vi "Config Core.vi"(8 "Error In":errorcluster, 10 "IConfigIn":refnum<class "IConfig.lvclass">, 11 "HardwareIn":refnum<class "IReference.lvclass">) -> (0 "Error Out":errorcluster, 2 "IConfigOut":refnum<class "IConfig.lvclass">, 3 "HardwareOut":refnum<class "IReference.lvclass">)   [LabVIEW 2019, in "IConfig.lvclass"]
uses:
  IConfig.lvclass
  IReference/IReference.lvclass
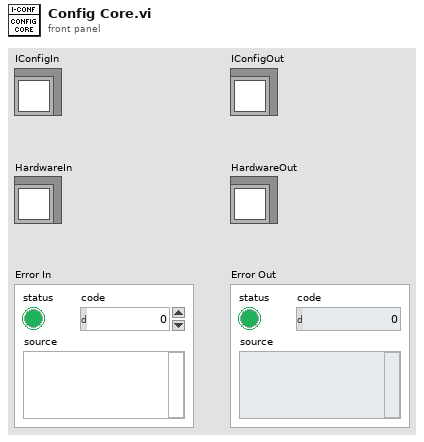
[diagram p1: front panel]
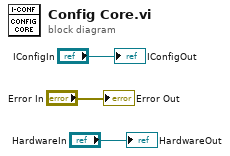
[diagram p0: block diagram]
diagram:
  "IConfigOut" <- "IConfigIn"
  "Error Out" <- "Error In"
  "HardwareOut" <- "HardwareIn"
